vi "Flash FPGA.vi"(8 "Error In":errorcluster, 9 "Bit File Path":path, 10 "Device ID":u32, 11 "Device Name":string) -> (0 "Error Out":errorcluster)   [LabVIEW 2011, in "LVH-Adept.lvlib" / "DJTG.lvlib"]
uses:
  <vilib>/LabVIEW Hacker/Adept/Private/DJTG/DJTG.lvlib
  <vilib>/LabVIEW Hacker/Adept/Private/DJTG/Private/Type Defs/Error.ctl
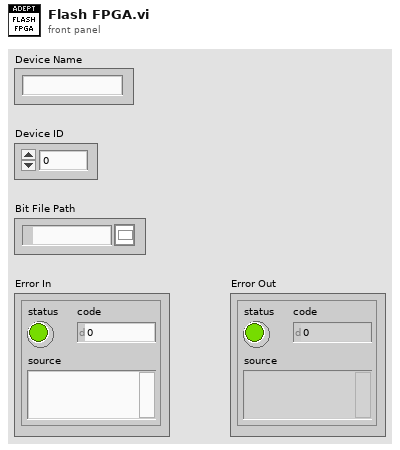
[diagram p1: front panel]
types:
  T1 = typedef "LVH-Adept.lvlib/DJTG.lvlib/Error.ctl" = enum16{"Unknown", "Enable", "PutTmsTdiBits", "GetTdoBits", "Disable", "Close", "Set Aux Reset", "Port Properties", "Get Speed", "Set Speed", "Get Port Count", "Get Batch Properties", "Enable Port", "Set Tmd Tdi Tck", "Get Tms Tdi Tdo Tck", "Put Tdi Bits", "Put Tms Bits", "Clock Tck", "Wait", "Batch", "Flash FPGA"}
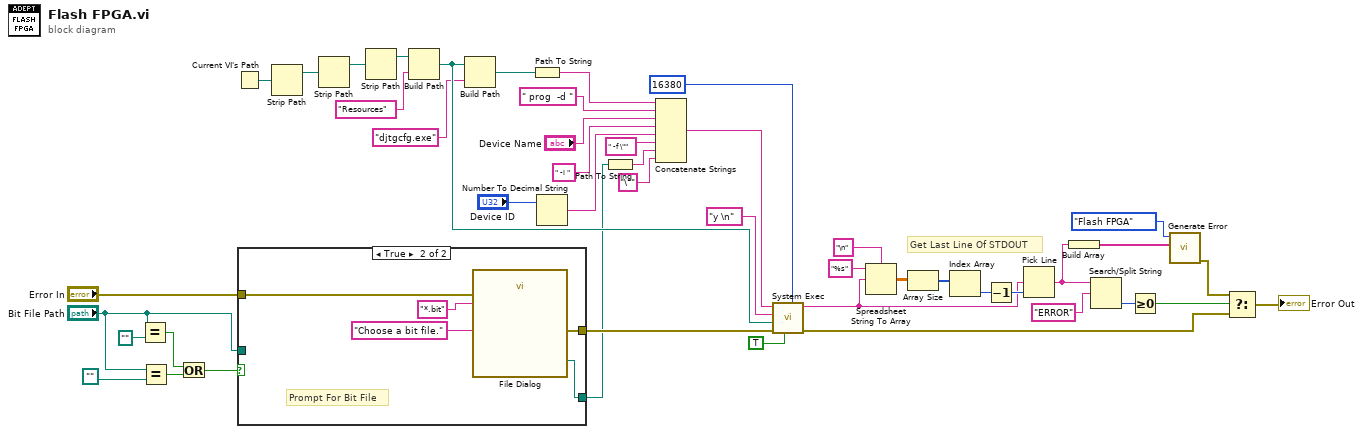
[diagram p0: block diagram]
diagram:
  # "Get Last Line Of STDOUT"
  n1 = Equal?(x="Bit File Path", y=path "") -> (x = y?=w23:bool)
  n2 = Equal?(x="Bit File Path", y=path "") -> (x = y?=w21:bool)
  n3 = Or(x=w23, y=w21) -> (x .or. y?=w20:bool)
  n4 = Current VI's Path() -> (path=w46:path)
  n5 = case shown="True" w20 {
    tunnel: [w48 w49] -> w18
    tunnel: "Error In" -> [w47 w52]
    tunnel: [w47 w51] -> w25
    tunnel: "Bit File Path" -> [w48 _]
    frame False {
      # "User Specified Bit File"
    }
    frame True {
      # "Prompt For Bit File"
      n6 = call "File Dialog"("prompt"="Choose a bit file." ("pattern (all files)"), "error in"=w52, "pattern (all files)"="*.bit") -> ("selected path"=w49:path, "error out"=w51:errorcluster)  [unwired: 9 in, 2 out]
    }
  }
  n7 = Strip Path(path=w46) -> (stripped path=w45:path)  [unwired: 1 out]
  n8 = Strip Path(path=w45) -> (stripped path=w44:path)  [unwired: 1 out]
  n9 = Strip Path(path=w44) -> (stripped path=w43:path)  [unwired: 1 out]
  n10 = Build Path(base path=w43, name or relative path="Resources") -> (appended path=w40:path)
  n11 = Build Path(base path=w40, name or relative path="djtgcfg.exe") -> (appended path=w38:path)
  n12 = Path To String(path=w38) -> (string=w37:string)
  n13 = Number To Decimal String(number="Device ID") -> (decimal integer string=w32:string)  [unwired: 1 in]
  n14 = Path To String(path=w18) -> (string=w29:string)
  n15 = Concatenate Strings(w37, " prog  -d " ("standard input"), "Device Name", " -i " ("standard input"), w32, " -f \"" ("standard input"), w29, "\"" ("standard input")) -> (w35:string)
  n16 = call <vilib>:"System Exec.vi"("expected output size  (4096)"=u32 16380, "run minimized? (F)"=TRUE, "error in (no error)"=w25, "working directory"=w40, "standard input"="y \n", "command line"=w35) -> ("error out"=w5:errorcluster, "standard output"=w11:string)  [unwired: 2 in, 2 out]
  n17 = Spreadsheet String To Array(delimiter (Tab)="\n" ("format string"), format string="%s", spreadsheet string=w11) -> (array=w15:dbl[][])  [unwired: 1 out]
  n18 = Array Size(array=w15) -> (size(s)=w14:i32[])
  n19 = Index Array(array=w14) -> (element=w13:i32)  [unwired: 1 in]
  n20 = Decrement(x=w13) -> (x-1=w12:i32)
  n21 = Pick Line(multi-line string=w11, line index=w12) -> (output string=w3:string)  [unwired: 1 in]
  n22 = Build Array(w3) -> (w2:string[])
  n23 = Search/Split String(string=w3, search string/char (-)="ERROR") -> (offset of match=w8:i32)  [unwired: 1 in, 2 out]
  n24 = Greater Or Equal To 0?(x=w8) -> (x >= 0?=w7:bool)
  n25 = call <vilib>:"Generate Error.vi"("Arguments"=w2, "DJTG Error"=Error."Flash FPGA") -> ("Error Out"=w6:errorcluster)  [unwired: 9 in]
  n26 = Select(t=w6, s=w7, f=w5) -> (s? t:f=→"Error Out":errorcluster)
